vi "Tug Motors.vi"(8 "error in (no error)":errorcluster, 9 "Prop Speed":dbl, 10 "MotorStop":bool, 11 "Rud Angle":dbl) -> (0 "error out":errorcluster)   [LabVIEW 2014]
uses:
  <vilib>/myRIO/Instrument Drivers/Onboard IO/PWM/typedefs/PWM Reference.ctl
  <vilib>/myRIO/Common/Instrument Driver Framework/Utilities/typedefs/myRIO Generic Hardware Reference.ctl
  <vilib>/myRIO/Common/Instrument Driver Framework/Utilities/typedefs/Hardware Version Enum.ctl
  <vilib>/myRIO/Common/Instrument Driver Framework/Utilities/typedefs/myRIO v1.0 Reference.ctl
  <vilib>/myRIO/Common/Instrument Driver Framework/Utilities/typedefs/Generic FPGA Reference.ctl
  <vilib>/myRIO/Common/Instrument Driver Framework/myRIO v1.0/PWM/typedefs/PWM Channels Enum.ctl
  <vilib>/myRIO/Instrument Drivers/Onboard IO/PWM/typedefs/PWM Configuration.ctl
  <vilib>/userdefined/High Color/nirio_resource_hc.ctl
  <vilib>/myRIO/Common/Instrument Driver Framework/Utilities/vis/Is FPGA Ref Available.vi
  <vilib>/myRIO/Common/Instrument Driver Framework/myRIO v1.0/PWM/vis/myRIO v1.1 Open PWM.vi
  <vilib>/myRIO/Instrument Drivers/Onboard IO/PWM/vis/Set Duty Cycle and Frequency.vi
  <vilib>/myRIO/Common/Instrument Driver Framework/Utilities/vis/Validate Channels.vi
  <vilib>/myRIO/Common/Instrument Driver Framework/myRIO v1.0/PWM/vis/myRIO v1.0 Reserve PWM.vi
  <vilib>/myRIO/Common/Instrument Driver Framework/myRIO v1.0/PWM/vis/myRIO v1.0 Build MUX Configuration PWM.vi
  <vilib>/myRIO/Common/Instrument Driver Framework/myRIO v1.0/Resource Manager/vis/myRIO v1.0 Reserve Channel List.vi
  <vilib>/myRIO/Common/Instrument Driver Framework/myRIO v1.0/Resource Manager/vis/myRIO v1.0 Create Configuration List.vi
  <vilib>/myRIO/Common/Instrument Driver Framework/myRIO v1.0/Resource Manager/vis/myRIO v1.0 Reserve Channel.vi
  <vilib>/myRIO/Common/Instrument Driver Framework/myRIO v1.0/Resource Manager/vis/myRIO v1.0 Unreserve Channel.vi
  <vilib>/myRIO/Common/Instrument Driver Framework/myRIO v1.0/Resource Manager/vis/myRIO v1.0 Build Mutex Name.vi
  <vilib>/Utility/VariantDataType/GetNumericInfo.vi
  <vilib>/Utility/error.llb/Error Cluster From Error Code.vi
  <vilib>/myRIO/Common/Instrument Driver Framework/myRIO v1.0/myRIO v1.1 Open.vi
  <vilib>/myRIO/Common/Instrument Driver Framework/Utilities/vis/IO Manager.vi
  <vilib>/myRIO/Common/Instrument Driver Framework/Utilities/vis/Configuration Manager.vi
  <vilib>/myRIO/Common/Instrument Driver Framework/myRIO v1.0/Resource Manager/vis/myRIO v1.0 Configure IO.vi
  <vilib>/myRIO/Common/Instrument Driver Framework/myRIO v1.0/myRIO v1.0 Close.vi
  <vilib>/myRIO/Common/Instrument Driver Framework/myRIO v1.0/PWM/vis/myRIO v1.0 Write PWM.vi
  <vilib>/myRIO/Express VI/Onboard IO/PWM/PWM Express VI.xnode
  <vilib>/myRIO/Instrument Drivers/Onboard IO/PWM/vis/myRIO PWM Open.xnode
  <vilib>/myRIO/Instrument Drivers/Onboard IO/PWM/PWM.lvlib
panel:
  # "This subVi sets the \nRudder angle and\nPropellor speed"
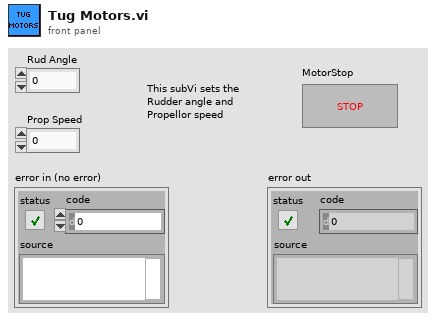
[diagram p1: front panel]
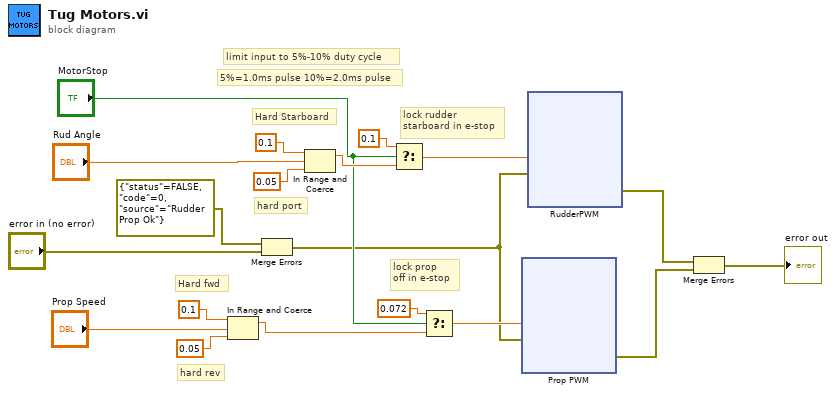
[diagram p0: block diagram]
diagram:
  # "lock prop \noff in e-stop"
  # "Hard fwd"
  # "hard rev"
  # "lock rudder \nstarboard in e-stop"
  # "5%=1.0ms pulse 10%=2.0ms pulse"
  # "Hard Starboard"
  # "hard port"
  # "limit input to 5%-10% duty cycle"
  n1 = In Range and Coerce(upper limit=0.1, x="Prop Speed", lower limit=0.05) -> (coerced(x)=w9:dbl)  [unwired: 1 out]
  n2 = Merge Errors "Merge Errors"(errorcluster {"status"=FALSE, "code"=0, "source"="Rudder Prop Ok"} ("error in (no error)"), "error in (no error)") -> (w1:errorcluster)
  n3 = In Range and Coerce(upper limit=0.1, x="Rud Angle", lower limit=0.05) -> (coerced(x)=w15:dbl)  [unwired: 1 out]
  n4 = Select(t=0.1, s="MotorStop", f=w15) -> (s? t:f=w16:dbl)
  n5 = Select(t=0.072, s="MotorStop", f=w9) -> (s? t:f=w4:dbl)
  n6 = xnode "Prop PWM"("Duty Cycle"=w4, "error in (no error)"=w1) -> ("error out"=w12:errorcluster)
  n7 = xnode "RudderPWM"("Duty Cycle"=w16, "error in (no error)"=w1) -> ("error out"=w13:errorcluster)
  n8 = Merge Errors "Merge Errors"(w13, w12) -> (→"error out":errorcluster)
